vi "Queue Init.vi"(9 "Queue Self":map{string, refnum<data-value>}(c390), 10 "Queue Caller":map{string, refnum<data-value>}(c390)) -> (3 "Base Queue Actor out":refnum<class "Base Queue Actor.lvclass">)   [LabVIEW 2021, in "jettl.lvlib" / "Base Queue Actor.lvclass"]
uses:
  Base Queue Actor.lvclass
  Msg/Msg/Msg.lvclass
  Queue State/Nominal Queue State/Nominal Queue State.lvclass
  C:/git/jettl/src/jettl/Queue State/Queue State/Queue State.lvclass
  Base Queue Actor.lvclass/Base Queue Actor.ctl
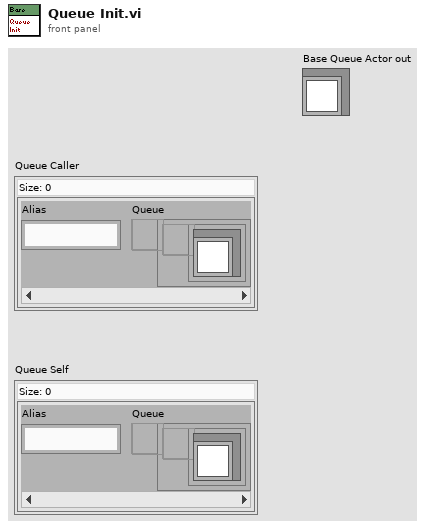
[diagram p1: front panel]
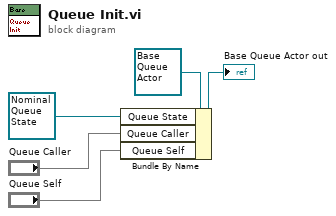
[diagram p0: block diagram]
diagram:
  n1 = Bundle By Name(cluster=refnum<class "Base Queue Actor.lvclass"> refnum ("Self Actor in"), "Queue State"=refnum<class "Nominal Queue State.lvclass"> refnum ("jettl.lvlib:Nominal Queue State.lvclass"), "Queue Caller"="Queue Caller", "Queue Self"="Queue Self") -> (→"Base Queue Actor out":refnum<class "Base Queue Actor.lvclass">)
